vi "Live window-Event handler-channel change.vi"(7 "Left/Right":T1) -> (0 "error out":errorcluster)   [LabVIEW 2020]
uses:
  Typedefs/Left-Right enum.ctl
  Globals/gl_Windows Ctrl refs.vi
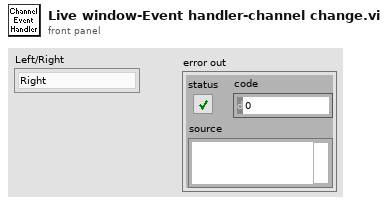
[diagram p1: front panel]
types:
  T1 = typedef "Left-Right enum.ctl" = enum16{"Right", "Left"}
  T2 = typedef "Live window-ctrl refs.ctl" = cluster{"This VI":refnum<vi>, "Pane":refnum<vi>, "Show REF Image Left":refnum<vi>, "Show REF Image Right":refnum<vi>, "Snapshot":refnum<vi>, "Left Image Palette":refnum<vi>, "Right Image Palette":refnum<vi>, "Left Channel":refnum<vi>, "Right Channel":refnum<vi>, "Left image intensity":refnum<vi>, "Right image intensity":refnum<vi>, "Left Image Display":T3, "Right Image Display":T3, "Refresh rate ind (Hz)":refnum<vi>, "Acq rate ind (Hz)":refnum<vi>, "Stop (ind)":refnum<vi>}
  T3 = typedef "Image display ref.ctl" = refnum<vi>
  T4 = typedef "Channel Selector.ctl" = enum16{"Red Channel", "Green Channel", "Blended"}
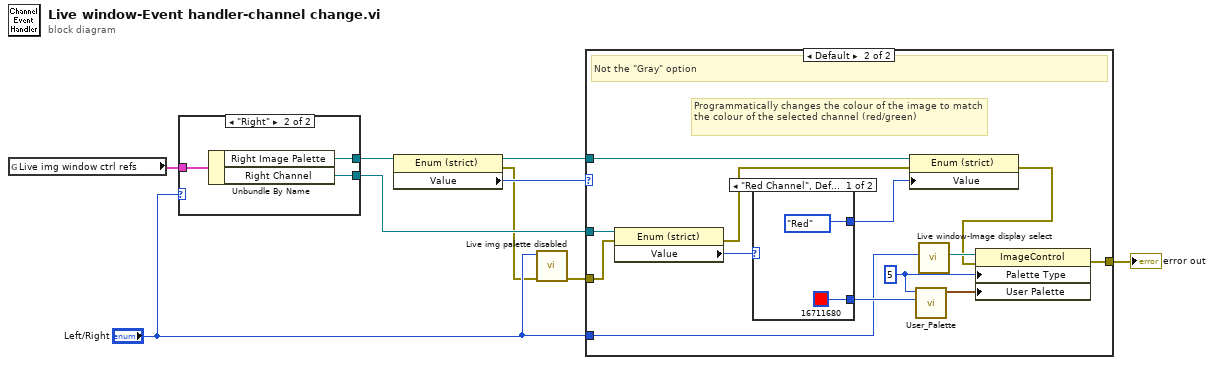
[diagram p0: block diagram]
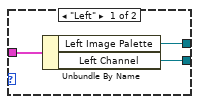
[diagram p2: hidden frame]
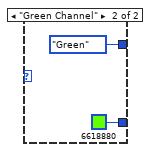
[diagram p4: hidden frame]
diagram:
  n1 = global read "gl_Windows Ctrl refs.vi" "Live img window ctrl refs"() -> (w6:T2)
  n2 = case shown="\"Right\"" "Left/Right" {
    tunnel: [w12 w15] -> w8
    tunnel: w6 -> [w11 w14]
    tunnel: [w10 w13] -> w3
    frame "Left" {
      n3 = Unbundle By Name(w11) -> ("Left Image Palette"=w12:refnum<vi>, "Left Channel"=w10:refnum<vi>)
    }
    frame "Right" {
      n4 = Unbundle By Name(w14) -> ("Right Image Palette"=w15:refnum<vi>, "Right Channel"=w13:refnum<vi>)
    }
  }
  n5 = property class="Enum (strict)"(reference=w8) -> (reference out=w9:refnum<vi>, error out=w2:errorcluster, "Value"=w7:enum16{"Gray", "Red", "Green"})  [unwired: 1 in]
  n6 = call "Live img palette disabled.vi"("error in (no error)"=w2, "Left/Right"="Left/Right") -> ("error out"=w1:errorcluster)  [unwired: 9 in]
  n7 = case shown="Default" w7 {
    tunnel: w9 -> [_ w25]
    tunnel: w3 -> [_ w22]
    tunnel: w1 -> [w16 w21]
    tunnel: [w16 w18] -> w5
    tunnel: "Left/Right" -> [_ w17]
    frame "Gray" {
    }
    frame Default {
      w27 = u32 5 ("t")
      # "Programmatically changes the colour of the image to match the colour of the selected channel (red/green)"
      # "Not the \"Gray\" option"
      n8 = property class="Enum (strict)"(reference=w22, error in=w21) -> (error out=w20:errorcluster, "Value"=w23:T4)  [unwired: 1 out]
      n9 = case shown="\"Red Channel\", Default" w23 {
        tunnel: [enum16{"Gray", "Red", "Green"}."Red" ("Left Image Palette") enum16{"Gray", "Red", "Green"}."Green" ("Left Image Palette")] -> w24
        tunnel: [u32 16711680 ("Color") u32 6618880 ("Color")] -> w28
        frame "Red Channel", Default {
        }
        frame "Green Channel" {
        }
      }
      n10 = property class="Enum (strict)"(reference=w25, error in=w20, "Value"=w24) -> (error out=w19:errorcluster)  [unwired: 1 out]
      n11 = call "User_Palette.vi"("Color"=w28, "Palette Number (gray)"=w27) -> ("Color Palette"=w29:cluster{"Red":u8, "Green":u8, "Blue":u8}[])  [unwired: 9 in]
      n12 = call "Live window-Image display select.vi"("Which image display?"=w17) -> ("Image display ref"=w26:T3)  [unwired: 10 in]
      n13 = property on="Property Node" class="ImageControl"(reference=w26, error in=w19, "Palette Type"=w27, "User Palette"=w29) -> (error out=w18:errorcluster)  [unwired: 1 out]
    }
  }
  "error out" <- w5
